vi "Servo_getAngle.vi"(3 "error in":errorcluster) -> (0 "error out":errorcluster, 1 "PWM10 Angle":dbl, 2 "PWM9 Angle":dbl)   [LabVIEW 2009, in "Servo.lvlib"]
doc: "Returns the current position of the camera, in the form of two angles."
uses:
  Servo.lvlib
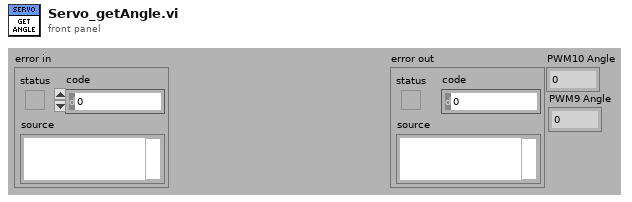
[diagram p1: front panel]
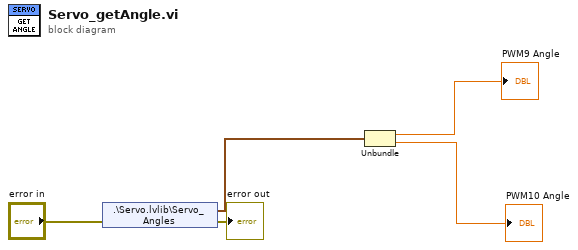
[diagram p0: block diagram]
diagram:
  n1 = shared-variable ".\\Servo.lvlib\\Servo_Angles"(error in="error in") -> (w3:cluster{"Angle in 3":dbl, "Angle in 3":dbl}, error out=→"error out":errorcluster)
  n2 = Unbundle(w3) -> ("Angle in 3"=→"PWM9 Angle":dbl, "Angle in 3"=→"PWM10 Angle":dbl)
